vi "getConnectionStatus.vi"(0 "SEDSpectrometer in":refnum<class "SEDSpectrometer.lvclass">, 1 "AvailableSpectrometer":u8[](array[numeric]), 2 "NumOfDevices":i32, 3 "error in (no error)":errorcluster) -> (7 "SEDSpectrometer out":refnum<class "SEDSpectrometer.lvclass">, 8 "DeviceStatus":string[][](table), 10 "error out":errorcluster)   [LabVIEW 2016, in "SEDSpectrometer.lvclass"]
uses:
  SEDSpectrometer.lvclass
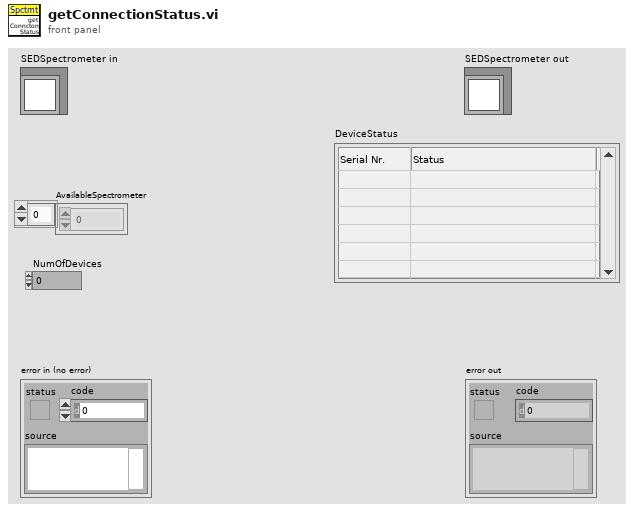
[diagram p1: front panel]
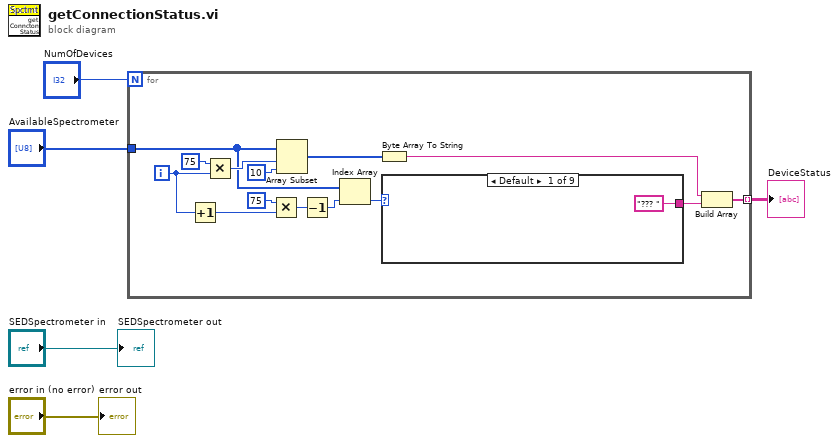
[diagram p0: block diagram]
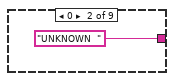
[diagram p2: hidden frame]
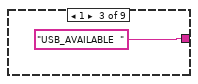
[diagram p3: hidden frame]
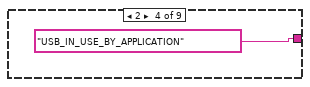
[diagram p4: hidden frame]
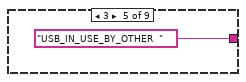
[diagram p5: hidden frame]
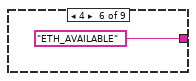
[diagram p6: hidden frame]
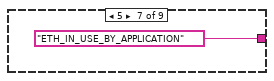
[diagram p7: hidden frame]
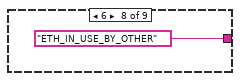
[diagram p8: hidden frame]
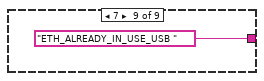
[diagram p9: hidden frame]
diagram:
  n1 = for {
    N: "NumOfDevices" -> [_]
    tunnel: "AvailableSpectrometer" -> [w11]
    tunnel: [w13] -> w1 mode=indexing
    i -> [w9]
    n2 = Increment(x=w9) -> (x+1=w8:i32)
    n3 = Multiply(x=75, y=w9) -> (x*y=w15:i32)
    n4 = Multiply(x=75, y=w8) -> (x*y=w7:i32)
    n5 = Array Subset(array=w11, index=w15, length=10) -> (w10:u8[])
    n6 = Decrement(x=w7) -> (x-1=w6:i32)
    n7 = Index Array(array=w11, index=w6) -> (element=w18:u8)
    n8 = Byte Array To String(unsigned byte array=w10) -> (string=w12:string)
    n9 = case shown="Default" w18 {
      tunnel: ["??? " "UNKNOWN  " "USB_AVAILABLE  " "USB_IN_USE_BY_APPLICATION" "USB_IN_USE_BY_OTHER  " "ETH_AVAILABLE" "ETH_IN_USE_BY_APPLICATION" "ETH_IN_USE_BY_OTHER" "ETH_ALREADY_IN_USE_USB "] -> w14
      frame Default {
      }
      frame 0 {
      }
      frame 1 {
      }
      frame 2 {
      }
      frame 3 {
      }
      frame 4 {
      }
      frame 5 {
      }
      frame 6 {
      }
      frame 7 {
      }
    }
    n10 = Build Array(w12, w14) -> (w13:string[])
  }
  "DeviceStatus" <- w1
  "error out" <- "error in (no error)"
  "SEDSpectrometer out" <- "SEDSpectrometer in"
